vi "a2ii.vi"() -> ()   [LabVIEW 2022 SP3]
uses:
  <vilib>/Skyline/Tag/Shared/typedefs/DataType.ctl
  <vilib>/numeric/Random Number (Range) DBL.vi
  <vilib>/Skyline/Configuration/Configuration HTTP_class/Open Configuration API Key.vi
  <vilib>/Skyline/Tag/Wrapper/Wrapper_class/Write Tag (DBL).vi
  <vilib>/Skyline/Tag/Wrapper/Wrapper_class/Close Tag (Single).vi
  <vilib>/Skyline/Configuration/Configuration HTTP_class/NI Skyline Configuration HTTP.lvclass
  <vilib>/Skyline/Tag/Wrapper/Wrapper HTTP_class/NI Skyline Tag HTTP.lvclass
  <vilib>/Skyline/Tag/Shared/NI Skyline Tag.lvlib
  <vilib>/Skyline/Tag/Wrapper/Wrapper_class/NI Skyline Tag.lvclass
panel:
  out "Random number":dbl
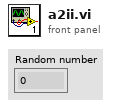
[diagram p1: front panel]
types:
  T1 = typedef "NI Skyline Tag.lvlib/DataType.ctl" = enum32{"Double", "I32", "String", "Boolean", "U64", "Timestamp"}
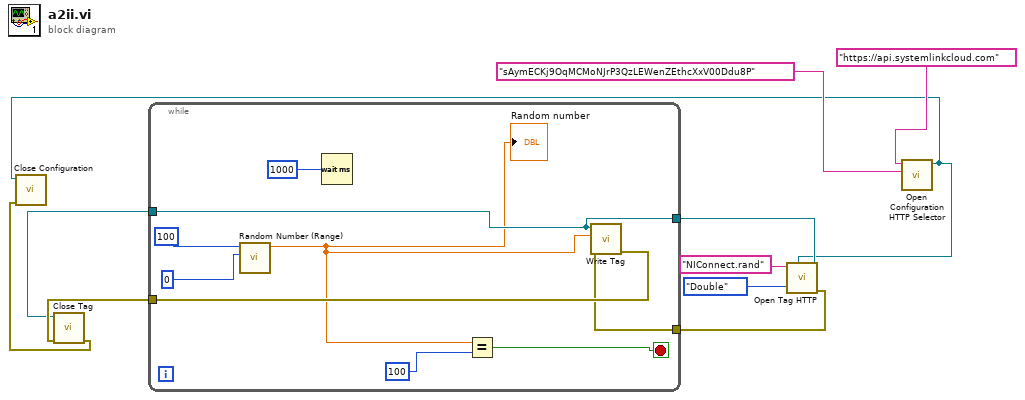
[diagram p0: block diagram]
diagram:
  n1 = call-poly <vilib>:"Open Configuration HTTP Selector.vi"("api key"="sAymECKj9OqMCMoNJrP3QzLEWenZEthcXxV00Ddu8P", "server url"="https://api.systemlinkcloud.com") -> ("configuration"=w1:refnum<class "NI Skyline Configuration HTTP.lvclass">)  [unwired: 8 in, 1 out]
  n2 = call <vilib>:"Open Tag HTTP.vi"("configuration"=w1, "Data Type"=DataType."Double", "path"="NIConnect.rand") -> ("error out"=w3:errorcluster, "tag"=w6:refnum<class "NI Skyline Tag.lvclass">)  [unwired: 7 in]
  n3 = while {
    tunnel: w6 -> [w13]
    tunnel: [w14] -> w5
    tunnel: [w13] -> w4
    tunnel: w3 -> [w12]
    stop <- w15 stop-if-true
    n4 = call-poly <vilib>:"Random Number (Range).vi"("lower bound (0)"=0, "upper bound (100)"=100) -> ("number"=w11:dbl)  [unwired: 9 in]
    "Random number" <- w11
    n5 = Wait (ms)(milliseconds to wait=u32 1000 ("millisecond timer value")) -> ()  [unwired: 1 out]
    n6 = Equal?(x=w11, y=100) -> (x = y?=w15:bool)
    n7 = call-poly <vilib>:"Write Tag.vi"("error in (no error)"=w12, "value"=w11, "tag in"=w13) -> ("error out"=w14:errorcluster)  [unwired: 7 in, 1 out]
  }
  n8 = call-poly <vilib>:"Close Tag.vi"("error in (no error)"=w5, "tag"=w4) -> ("error out"=w2:errorcluster)  [unwired: 9 in]
  n9 = call-dynamic "Close Configuration.vi"("error in (no error)"=w2, "configuration"=w1) -> ()  [unwired: 9 in, 1 out]
